vi "Get axis quick info.vi"(7 "path in":path, 8 "error in":errorcluster, 10 "deviceHandle":u64, 11 "Axis status in":T1 {"Index" items=["1", "2", "3"]; "ActuatorType" items=["Linear", "Rotator", "Goniometer"]}) -> (0 "error out":errorcluster, 1 "axis out":u8, 2 "deviceHandle out":u64, 3 "Axis status":T1 {"Index" items=["1", "2", "3"]; "ActuatorType" items=["Linear", "Rotator", "Goniometer"]})   [LabVIEW 2022 SP3, in "SampleRotator.lvlib"]
doc: "Queries axis (actuator) status, actual position, and current settings of amplitude, frequency.\n\ninputs: \npath to DLL; handle; axis; error cluster\n\noutputs:\nhandle; axis; axis status; error cluster"
uses:
  SampleRotator.lvlib
  ctl/Axis status.ctl
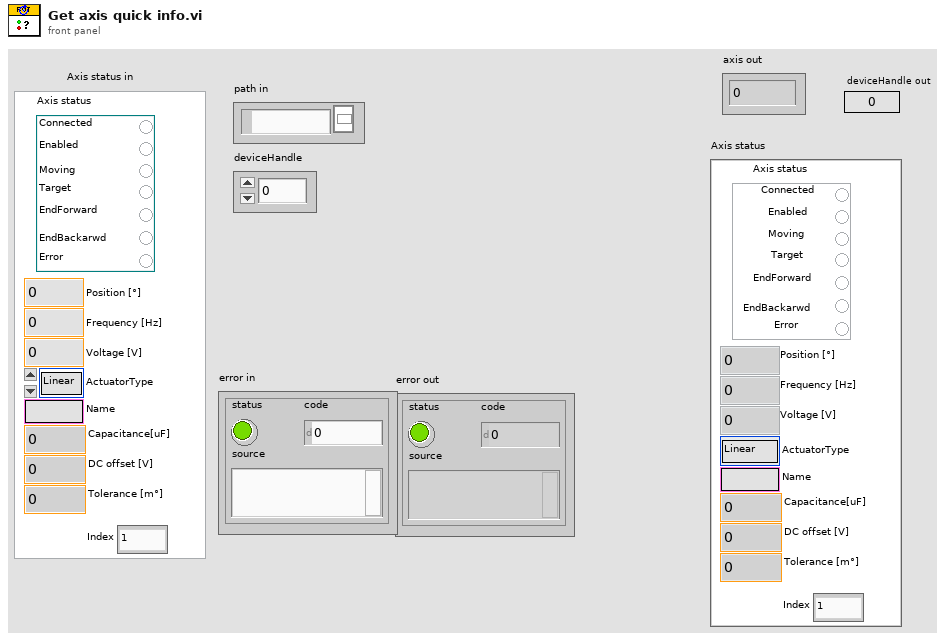
[diagram p1: front panel]
types:
  T1 = typedef "SampleRotator.lvlib/Axis status.ctl" = cluster{"Axis status":cluster{"Connected":bool, "Enabled":bool, "Moving":bool, "Target":bool, "EndForward":bool, "EndBackarwd":bool, "Error":bool}, "Position [°]":dbl, "Frequency [Hz]":dbl, "Voltage [V]":dbl, "Capacitance[uF]":dbl, "Name":string, "ActuatorType":u16, "DC offset [V]":dbl, "Tolerance [m°]":dbl, "Index":u8}
  T2 = cluster{"connected":bool, "enabled":bool, "moving":bool, "target":bool, "EotFwd":bool, "EotBwd":bool, "error":bool}
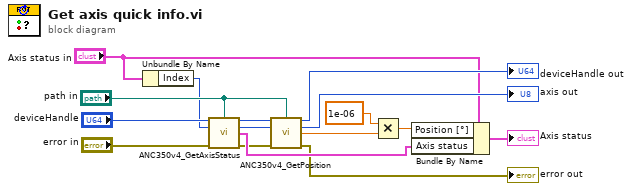
[diagram p0: block diagram]
diagram:
  n1 = Unbundle By Name("Axis status in") -> ("Index"=w1:u8)
  n2 = call <instrlib>:"ANC350v4_GetAxisStatus.vi"("deviceHandle"="deviceHandle", "Path to *.DLL"="path in", "axis"=w1, "error in"="error in") -> ("deviceHandle"=w12:u64, "axis"=w11:u8, "Axis status"=w13:T2, "error ANC350v4_getAxisStatus"=w10:errorcluster)  [unwired: 7 in, 1 out]
  n3 = call <instrlib>:"ANC350v4_GetPosition.vi"("deviceHandle"=w12, "Path to *.DLL"="path in", "axis"=w11, "error in"=w10) -> ("deviceHandle"=→"deviceHandle out":u64, "axis"=→"axis out":u8, "Position [µm | m°]"=w15:dbl, "error ANC350v4_getPosition"=→"error out":errorcluster)  [unwired: 8 in]
  n4 = Multiply(x=1e-06, y=w15) -> (x*y=w9:dbl)
  n5 = Bundle By Name(cluster="Axis status in", "Position [°]"=w9, "Axis status"=w13) -> (→"Axis status":T1)
